vi "Load_Source_Type.vi"(8 "error in (no error)":errorcluster, 9 "index in":string, 11 "buildObject":T1) -> (0 "error out":errorcluster, 1 "index out":string, 3 "IB_Source out":refnum<class "IB_Source.lvclass">)   [LabVIEW 2020, in "IB_Source.lvclass"]
uses:
  <vilib>/AppBuilder/IB_Classes/Source/IB_Source.lvclass
  <vilib>/AppBuilder/IB_Classes/Source/IB_Source.lvclass/IB_Source.ctl
  <vilib>/AppBuilder/IB_Classes/Source/Container/Folder/IB_Source_Folder.lvclass
  <vilib>/AppBuilder/IB_Classes/Source/File/IB_Source_File.lvclass
  <vilib>/AppBuilder/IB_Classes/Source/Container/Build/SDIST/IB_SDIST.lvclass
  <vilib>/AppBuilder/IB_Classes/Source/Container/Build/DLL/IB_DLL.lvclass
  <vilib>/AppBuilder/IB_Classes/Source/Container/Build/EXE/IB_EXE.lvclass
  <vilib>/AppBuilder/IB_Classes/Source/Container/Build/CGen/IB_CGen.lvclass
  <vilib>/AppBuilder/IB_Classes/Source/Container/Build/NET/IB_DotNET.lvclass
  <vilib>/AppBuilder/IB_Classes/Source/Container/Build/PackedLib/IB_PackedLib.lvclass
  <vilib>/AppBuilder/IB_Classes/Source/Container/Build/RestfulWS/IB_RestfulWS.lvclass
  e:/builds/penguin/labview/branches/2020/dev/dist/vi.lib/AppBuilder/IB_Classes/Source/Container/IB_Source_Container.lvclass
  e:/builds/penguin/labview/branches/2020/dev/dist/vi.lib/AppBuilder/IB_Classes/Source/IB_Source.lvclass
  e:/builds/penguin/labview/branches/2020/dev/dist/vi.lib/AppBuilder/IB_Classes/Source/Container/Folder/IB_Source_Folder.lvclass
  e:/builds/penguin/labview/branches/2020/dev/dist/vi.lib/AppBuilder/IB_Classes/Source/File/IB_Source_File.lvclass
  e:/builds/penguin/labview/branches/2020/dev/dist/vi.lib/AppBuilder/IB_Classes/Source/Container/Build/IB_Source_Build.lvclass
  e:/builds/penguin/labview/branches/2020/dev/dist/vi.lib/AppBuilder/IB_Classes/Source/Container/Build/SDIST/IB_SDIST.lvclass
  e:/builds/penguin/labview/branches/2020/dev/dist/vi.lib/AppBuilder/IB_Classes/Source/Container/Build/DLL/IB_DLL.lvclass
  e:/builds/penguin/labview/branches/2020/dev/dist/vi.lib/AppBuilder/IB_Classes/Source/Container/Build/EXE/IB_EXE.lvclass
  e:/builds/penguin/labview/branches/2020/dev/dist/vi.lib/AppBuilder/IB_Classes/Source/Container/Build/RestfulWS/IB_RestfulWS.lvclass
  e:/builds/penguin/labview/branches/2020/dev/dist/vi.lib/AppBuilder/IB_Classes/Source/Container/Build/PackedLib/IB_PackedLib.lvclass
  e:/builds/penguin/labview/branches/2020/dev/dist/vi.lib/AppBuilder/IB_Classes/Source/Container/Build/NET/IB_DotNET.lvclass
  e:/builds/penguin/labview/branches/2020/dev/dist/vi.lib/AppBuilder/IB_Classes/Source/Container/Build/CGen/IB_CGen.lvclass
  <resource>/Framework/Providers/API/ItemRef.ctl
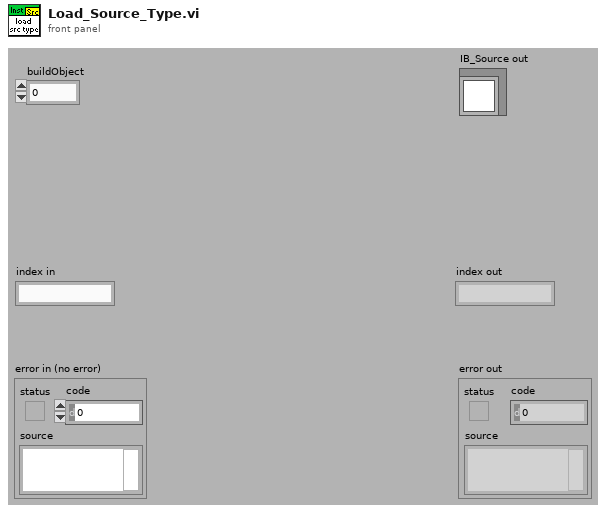
[diagram p1: front panel]
types:
  T1 = typedef "ItemRef.ctl" = u64
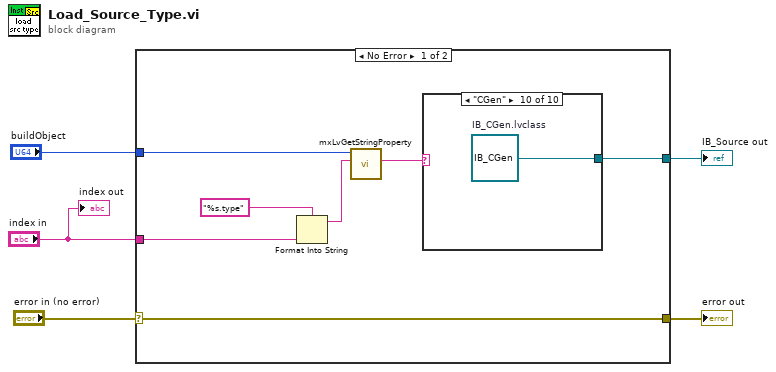
[diagram p0: block diagram]
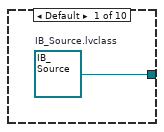
[diagram p2: hidden frame]
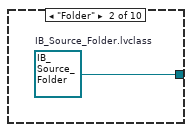
[diagram p3: hidden frame]
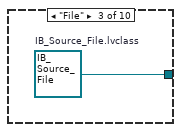
[diagram p4: hidden frame]
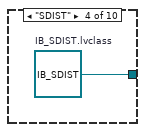
[diagram p5: hidden frame]
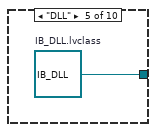
[diagram p6: hidden frame]
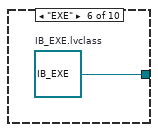
[diagram p7: hidden frame]
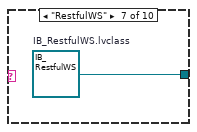
[diagram p8: hidden frame]
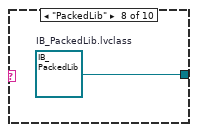
[diagram p9: hidden frame]
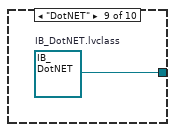
[diagram p10: hidden frame]
diagram:
  n1 = case shown="No Error" "error in (no error)" {
    selector: "error in (no error)" -> [w12 w23]
    tunnel: [w12 w23] -> w4
    tunnel: [w7 _] -> w3
    tunnel: "buildObject" -> [w8 _]
    tunnel: "index in" -> [w6 _]
    frame No Error {
      n2 = Format Into String(format string="%s.type", w6) -> (resulting string=w10:string)  [unwired: 2 in, 1 out]
      n3 = call <resource>:"mxLvGetStringProperty.vi"("Tag"=w10, "Item"=w8) -> ("Value"=w11:string)  [unwired: 1 in, 8 out]
      n4 = case shown="\"CGen\"" w11 {
        tunnel: [w13 w14 w15 w16 w17 w18 w19 w20 w21 w22] -> w7
        frame Default {
          w13 = refnum<class "IB_Source.lvclass"> refnum  # IB_Source.lvclass
        }
        frame "Folder" {
          w14 = refnum<class "IB_Source_Folder.lvclass"> refnum  # IB_Source_Folder.lvclass
        }
        frame "File" {
          w15 = refnum<class "IB_Source_File.lvclass"> refnum  # IB_Source_File.lvclass
        }
        frame "SDIST" {
          w16 = refnum<class "IB_SDIST.lvclass"> refnum  # IB_SDIST.lvclass
        }
        frame "DLL" {
          w17 = refnum<class "IB_DLL.lvclass"> refnum  # IB_DLL.lvclass
        }
        frame "EXE" {
          w18 = refnum<class "IB_EXE.lvclass"> refnum  # IB_EXE.lvclass
        }
        frame "RestfulWS" {
          w19 = refnum<class "IB_RestfulWS.lvclass"> refnum  # IB_RestfulWS.lvclass
        }
        frame "PackedLib" {
          w20 = refnum<class "IB_PackedLib.lvclass"> refnum  # IB_PackedLib.lvclass
        }
        frame "DotNET" {
          w21 = refnum<class "IB_DotNET.lvclass"> refnum  # IB_DotNET.lvclass
        }
        frame "CGen" {
          w22 = refnum<class "IB_CGen.lvclass"> refnum  # IB_CGen.lvclass
        }
      }
    }
    frame Error {
    }
  }
  "error out" <- w4
  "IB_Source out" <- w3
  "index out" <- "index in"
